vi "LoadComplexArrayFromFile.vi"(8 "error in":errorcluster, 11 "SourceFileName":string) -> (0 "error out":errorcluster, 3 "Array":csg[](array[numeric]))   [LabVIEW 2014]
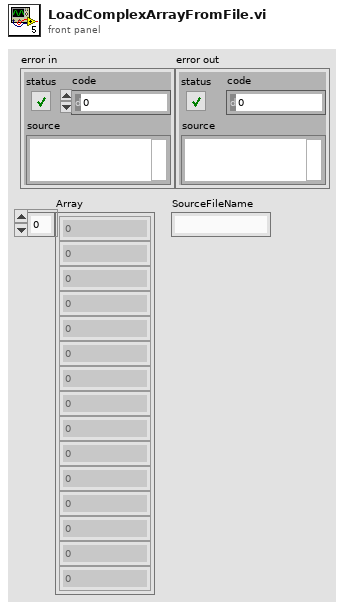
[diagram p1: front panel]
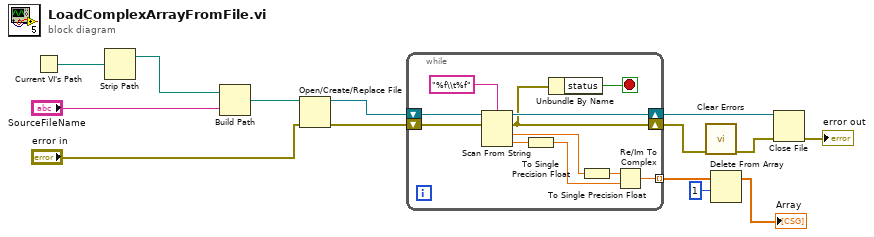
[diagram p0: block diagram]
diagram:
  n1 = Current VI's Path() -> (path=w7:path)
  n2 = Strip Path(path=w7) -> (stripped path=w6:path)  [unwired: 1 out]
  n3 = Build Path(base path=w6, name or relative path="SourceFileName") -> (appended path=w5:path)
  n4 = Open/Create/Replace File(file path (use dialog)=w5, error in="error in") -> (refnum out=w12:refnum<file>, error out=w11:errorcluster)  [unwired: 4 in, 1 out]
  n5 = while {
    shift-right: [w22] -> w9
    shift-left: w12 -> [w25]
    shift-right: [w18] -> w10
    shift-left: w11 -> [w24]
    tunnel: [w19] -> w4 mode=indexing
    stop <- w17 stop-if-true
    n6 = Scan From String("%f\\t%f" ("format string"), w25, w24) -> (w22:refnum<file>, w18:errorcluster, output 1=w21:dbl, output 2=w20:dbl)  [unwired: 2 in]
    n7 = To Single Precision Float(number=w20) -> (single precision float=w16:sgl)
    n8 = Unbundle By Name(w18) -> ("status"=w17:bool)
    n9 = To Single Precision Float(number=w21) -> (single precision float=w15:sgl)
    n10 = Re/Im To Complex(1:w16, 2:w15) -> (0:w19:csg)
  }
  n11 = call <vilib>:"Clear Errors.vi"("error in (no error)"=w10) -> ("error out"=w1:errorcluster)  [unwired: 5 in, 1 out]
  n12 = Delete From Array(array=w4, length=1) -> (array with subset deleted=→"Array":csg[])  [unwired: 1 in, 1 out]
  n13 = Close File(refnum=w9, error in=w1) -> (error out=→"error out":errorcluster)  [unwired: 1 out]
